vi "TestiLabviewLIVELowLevelv3 - Copy.vi"() -> ()   [LabVIEW 2018]
uses:
  <vilib>/myRIO/Instrument Drivers/Onboard IO/PWM/typedefs/PWM Reference.ctl
  <vilib>/myRIO/Common/Instrument Driver Framework/Utilities/typedefs/myRIO Generic Hardware Reference.ctl
  <vilib>/myRIO/Common/Instrument Driver Framework/Utilities/typedefs/Hardware Version Enum.ctl
  <vilib>/myRIO/Common/Instrument Driver Framework/Utilities/typedefs/myRIO v1.0 Reference.ctl
  <vilib>/myRIO/Common/Instrument Driver Framework/Utilities/typedefs/Generic FPGA Reference.ctl
  <vilib>/myRIO/Common/Instrument Driver Framework/myRIO v1.0/PWM/typedefs/PWM Channels Enum.ctl
  <vilib>/myRIO/Instrument Drivers/Onboard IO/PWM/typedefs/PWM Configuration.ctl
  <vilib>/userdefined/High Color/nirio_resource_hc.ctl
  <vilib>/vision/Image Controls.llb/IMAQ Image.ctl
  <vilib>/myRIO/Common/Instrument Driver Framework/myRIO v1.0/PWM/vis/myRIO v1.1 Open PWM.vi
  <vilib>/myRIO/Common/Instrument Driver Framework/Utilities/vis/Validate Channels.vi
  <vilib>/myRIO/Common/Instrument Driver Framework/myRIO v1.0/PWM/vis/myRIO v1.0 Reserve PWM.vi
  <vilib>/myRIO/Common/Instrument Driver Framework/myRIO v1.0/UART/vis/myRIO v1.0 Close UART.vi
  <vilib>/myRIO/Common/Instrument Driver Framework/myRIO v1.0/PWM/vis/myRIO v1.0 Build MUX Configuration PWM.vi
  <vilib>/myRIO/Common/Instrument Driver Framework/myRIO v1.0/Resource Manager/vis/myRIO v1.0 Reserve Channel List.vi
  <vilib>/myRIO/Common/Instrument Driver Framework/myRIO v1.0/Resource Manager/vis/myRIO v1.0 Create Configuration List.vi
  <vilib>/myRIO/Common/Instrument Driver Framework/myRIO v1.0/Resource Manager/vis/myRIO v1.0 Reserve Channel.vi
  <vilib>/myRIO/Common/Instrument Driver Framework/myRIO v1.0/Resource Manager/vis/myRIO v1.0 Unreserve Channel.vi
  <vilib>/myRIO/Common/Instrument Driver Framework/myRIO v1.0/Resource Manager/vis/myRIO v1.0 Build Mutex Name.vi
  <vilib>/Utility/VariantDataType/GetNumericInfo.vi
  <vilib>/Utility/error.llb/Error Cluster From Error Code.vi
  <vilib>/myRIO/Common/Instrument Driver Framework/myRIO v1.0/myRIO v1.1 Open.vi
  <vilib>/myRIO/Common/Instrument Driver Framework/Utilities/vis/IO Manager.vi
  <vilib>/myRIO/Common/Instrument Driver Framework/Utilities/vis/Configuration Manager.vi
  <vilib>/myRIO/Common/Instrument Driver Framework/myRIO v1.0/Resource Manager/vis/myRIO v1.0 Configure IO.vi
  <vilib>/myRIO/Common/Instrument Driver Framework/myRIO v1.0/myRIO v1.0 Close.vi
  <vilib>/myRIO/Common/Instrument Driver Framework/myRIO v1.0/PWM/vis/myRIO v1.0 Write PWM.vi
  <vilib>/myRIO/Common/Instrument Driver Framework/Utilities/vis/FPGA Ref Manager.vi
  <vilib>/myRIO/Common/Instrument Driver Framework/myRIO v1.0/myRIO v1.0 Reset FPGA.vi
  <vilib>/myRIO/Common/Instrument Driver Framework/myRIO v1.0/IRQ/vis/myRIO v1.0 IRQ Info FGV.vi
  <vilib>/myRIO/Common/Instrument Driver Framework/myRIO v1.0/IRQ/vis/myRIO v1.0 Timer IRQ Info FGV.vi
  <vilib>/myRIO/Common/Instrument Driver Framework/myRIO v1.0/IRQ/vis/myRIO v1.0 ISR Agent.vi
  <vilib>/myRIO/Instrument Drivers/Onboard IO/PWM/vis/myRIO PWM Open.xnode
  <vilib>/myRIO/Instrument Drivers/Onboard IO/PWM/PWM.lvlib
  <vilib>/myRIO/Instrument Drivers/Utilities/Utilities.lvlib
  <vilib>/vision/driver/NI_Vision_Acquisition_Software.lvlib
  <vilib>/vision/NI_Vision_Development_Module.lvlib
panel:
  in  "Number of Erosion (Advanced Morphology 1)":i32=12
  in  "Structuring Element (Basic Morphology 1) 2":i32[][](array[numeric])=[[0, 1, 0], [1, 1, 1], [0, 1, 0]]
  in  "Range (Threshold 1) 2":cluster{"Lower value":sgl, "Upper value":sgl}={"Lower value"=230.0, "Upper value"=255.0}
  in  "Color Plane (Color Plane Extraction 1) 2":i32(ring)=1 items=["Red", "Green", "Blue", "Hue", "Saturation", "Luminance", "Value", "Intensity"]
  in  "logfile base name":string="logfile"
  out "logfile name":path
  out "Image 5":T1(plugin-control)
  out "Antal isbjerg 4":i32
  out "X 4":dbl[](array[numeric])
  out "Y 4":dbl[](array[numeric])
  in  "Stop":bool
  # "Tager isbjerge i rækkefølgen: y: 0 -> max"
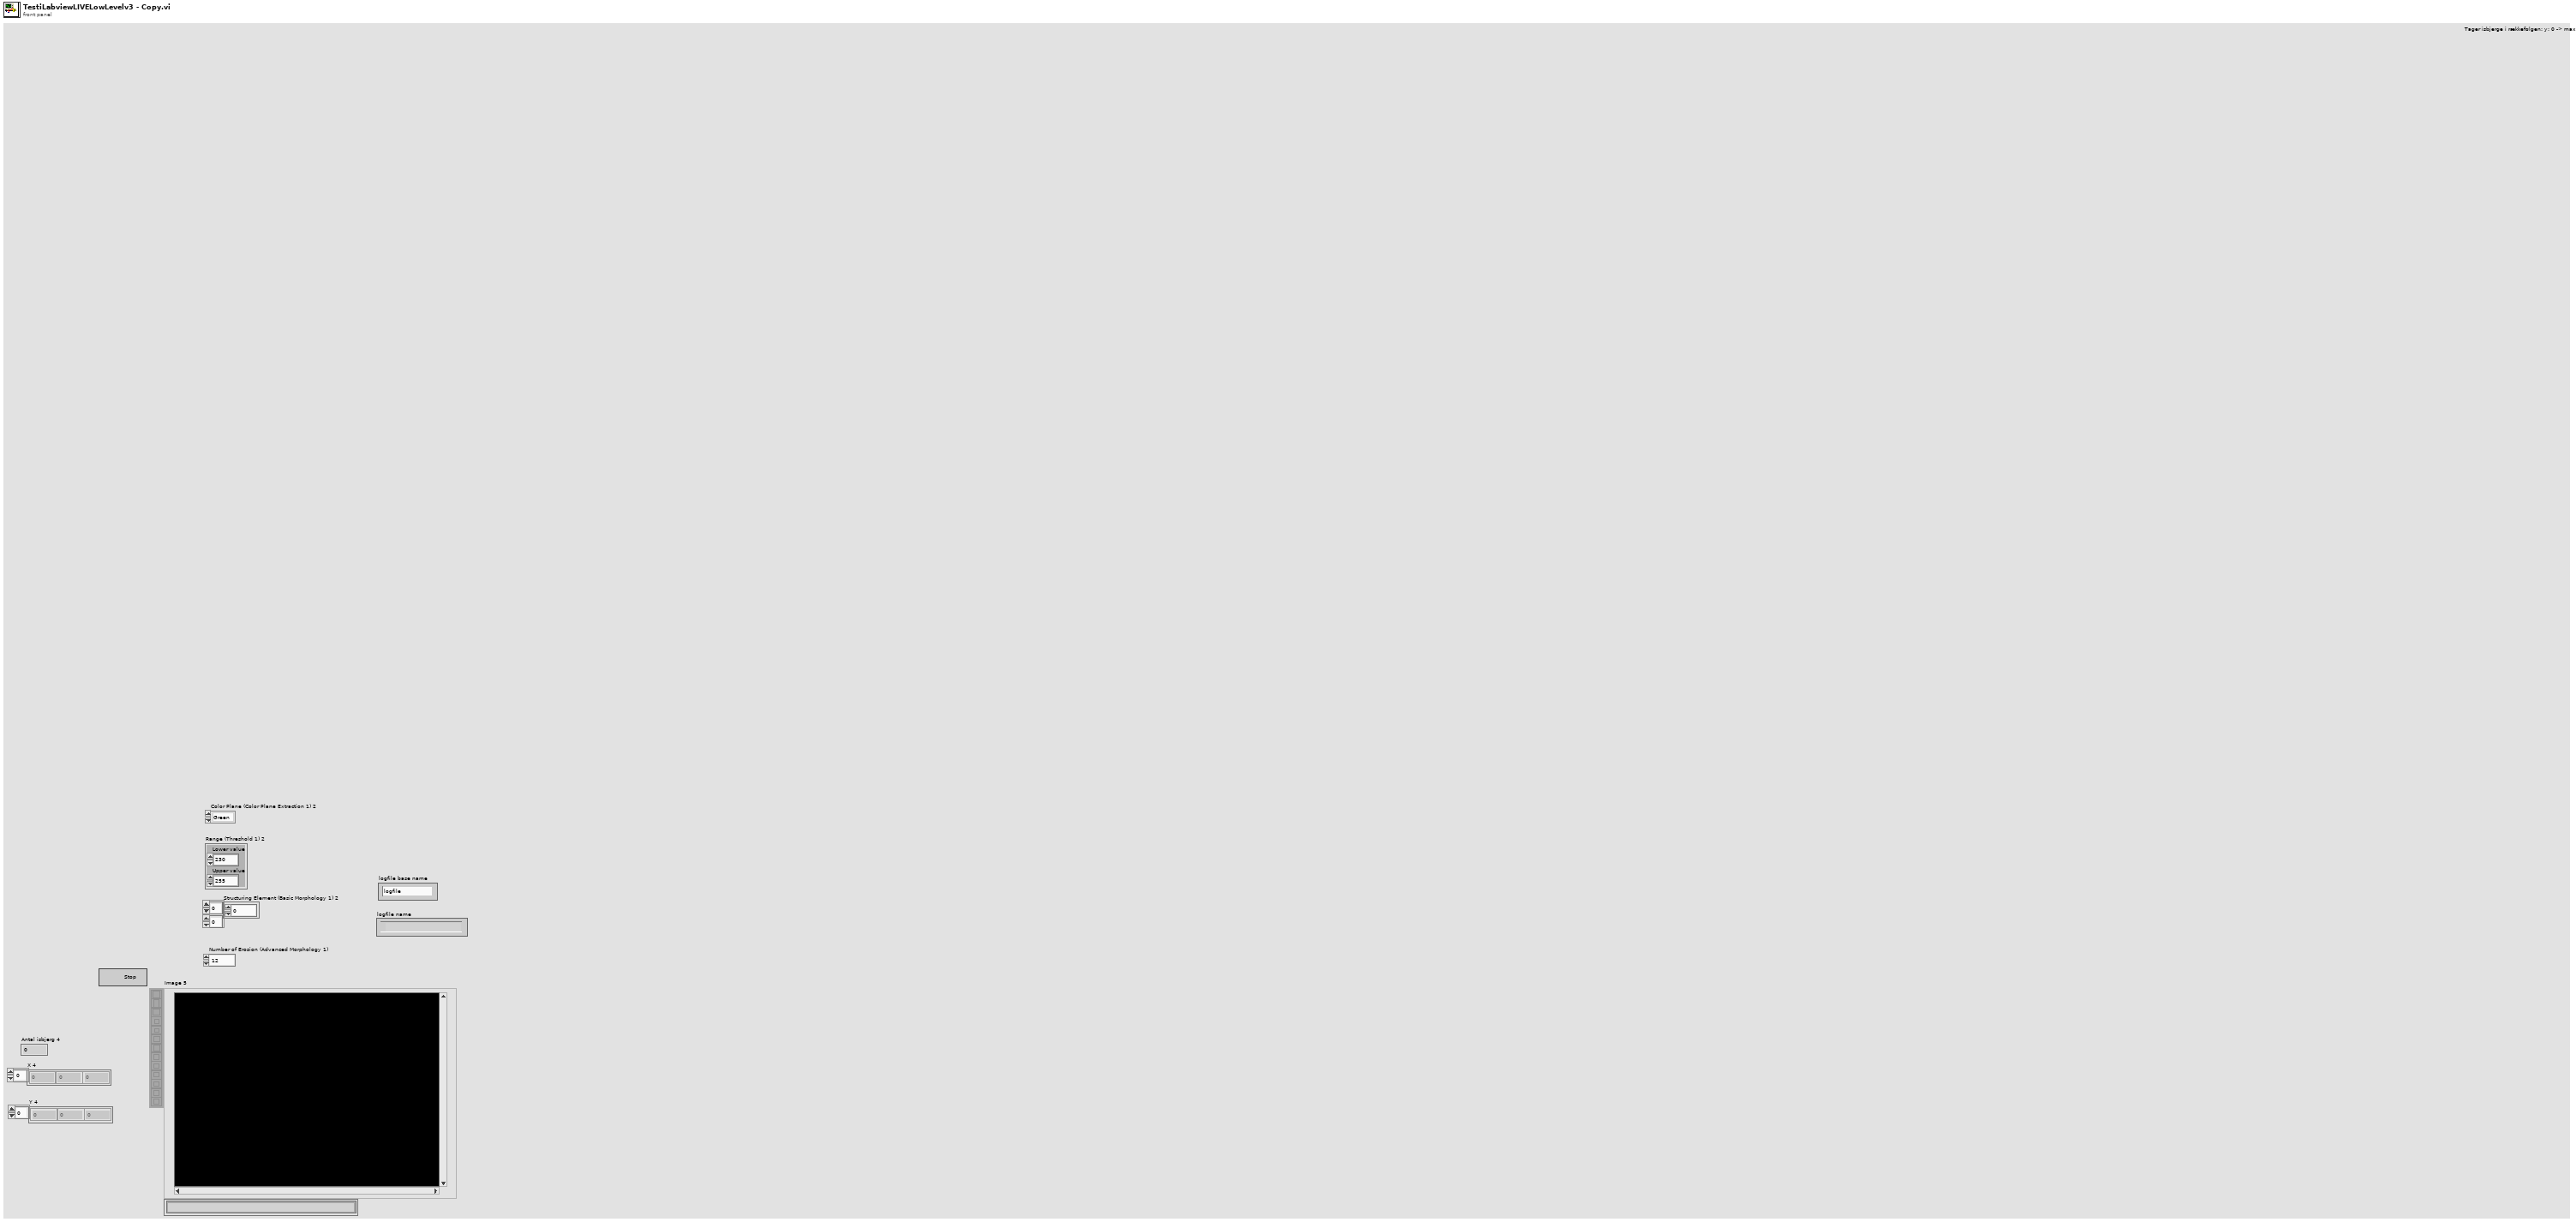
[diagram p1: front panel]
types:
  T1 = typedef "IMAQ Image.ctl" = refnum<image>
  T2 = typedef "nirio_resource_hc.ctl" = tag
  T3 = typedef "Hardware Version Enum.ctl" = enum16{"Unknown", "myRIO-1900", "myRIO-1950", "roboRIO", "NI ELVIS RIO CM", "ELVIS III"}
  T4 = enum32{"AutoM", "Close", "Dilate", "Erode", "Gradient", "Gradient out", "Gradient in", "Hit miss", "Open", "PClose", "POpen", "Thick", "Thin"}
  T5 = typedef "PWM.lvlib/PWM Reference.ctl" = cluster{"myRIO Reference":T6, "PWM Channels Enum":T9, "PWM Configuration":T10}
  T6 = typedef "myRIO Generic Hardware Reference.ctl" = cluster{"myRIO Model":T3, "myRIO Hardware Reference":T7}
  T7 = typedef "myRIO v1.0 Reference.ctl" = cluster{"Generic FPGA Reference":T8, "Allow multiple opens":bool}
  T8 = typedef "Generic FPGA Reference.ctl" = refnum<k20>
  T9 = typedef "PWM Channels Enum.ctl" = enum16{"Not Connected", "C/PWM0", "C/PWM1", "A/PWM0", "A/PWM1", "A/PWM2", "A/PWM3", "A/PWM4", "A/PWM5", "A/PWM6", "A/PWM7", "A/PWM8", "A/PWM9", "A/PWM10", "A/PWM11", "A/PWM12", "A/PWM13", "A/PWM14", "A/PWM15", "A/PWM16", "A/PWM17", "A/PWM18", "A/PWM19", "B/PWM0", "B/PWM1", "B/PWM2", "B/PWM3", "B/PWM4", "B/PWM5", "B/PWM6", "B/PWM7", "B/PWM8", "B/PWM9", "B/PWM10", "B/PWM11", "B/PWM12", "B/PWM13", "B/PWM14", "B/PWM15", "B/PWM16", "B/PWM17", "B/PWM18", "B/PWM19", "PWM/PWM0", "PWM/PWM1", "PWM/PWM2", "PWM/PWM3", "PWM/PWM4", "PWM/PWM5", "PWM/PWM6", "PWM/PWM7", "PWM/PWM8", "PWM/PWM9"}
  T10 = typedef "PWM.lvlib/PWM Configuration.ctl" = cluster{"Frequency":dbl, "Duty Cycle":dbl}
  T11 = typedef "Image Type" = u32
  T12 = typedef "IMAQdx.ctl" = refnum<k21>
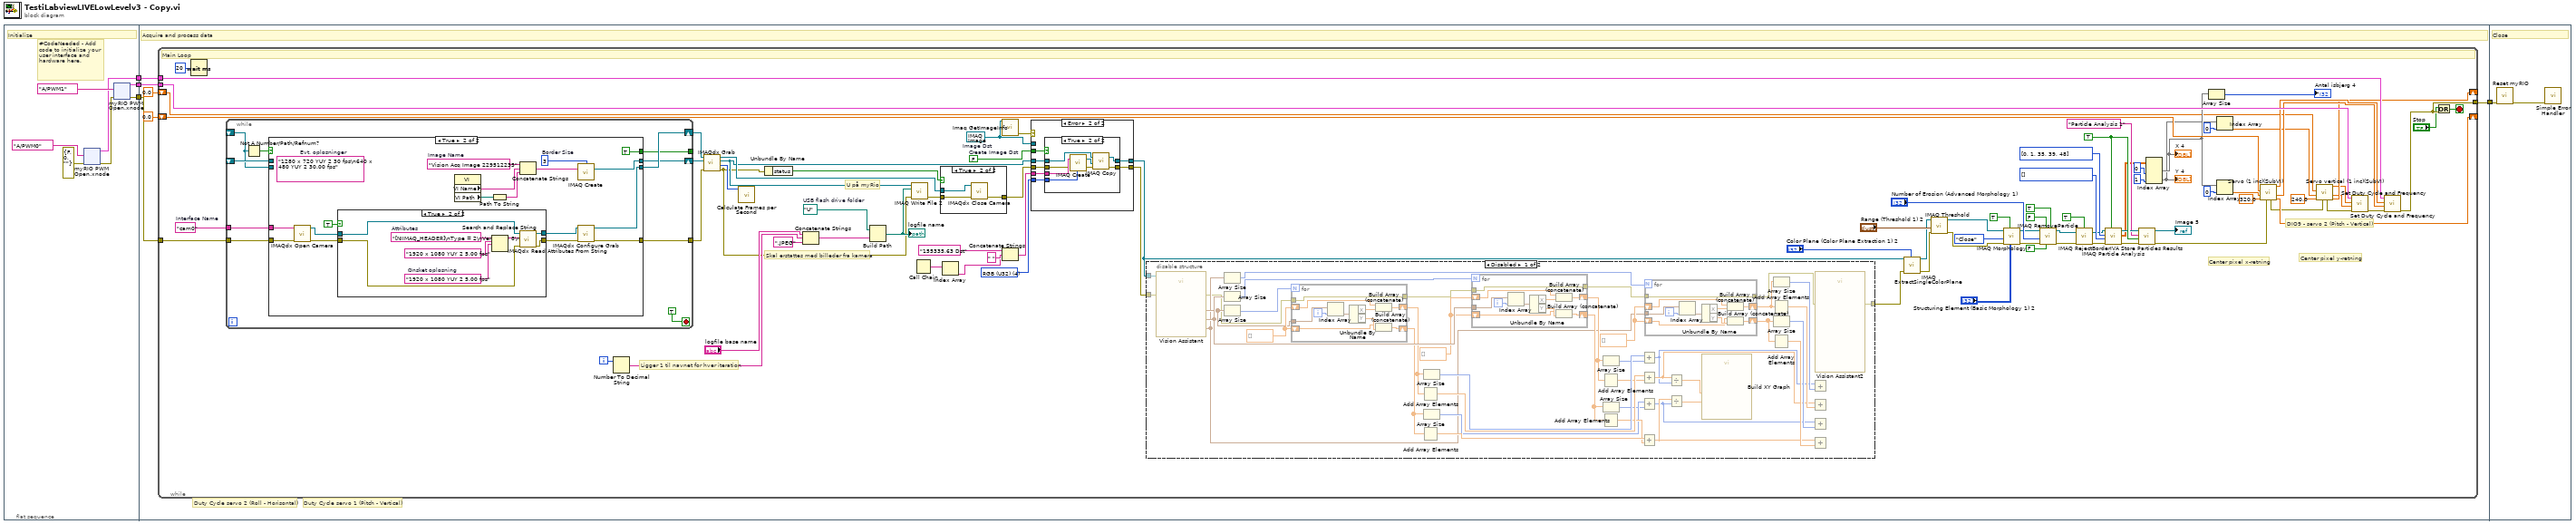
[diagram p0: block diagram]
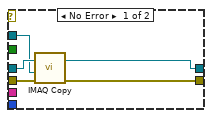
[diagram p6: hidden frame]
diagram:
  n1 = flat-sequence {
    tunnel: [w11] -> w4
    tunnel: [w10] -> w3
    tunnel: [w7] -> w2
    tunnel: w4 -> [w49]
    tunnel: w3 -> [w44]
    tunnel: w2 -> [w48]
    tunnel: [w47] -> w1
    tunnel: w1 -> [w278]
    frame #0 {
      # "#CodeNeeded - Add code to initialize your user interface and hardware here."
      # "Initialize"
      n2 = xnode "myRIO PWM Open.xnode"("error in (no error)"=errorcluster {"status"=FALSE, "code"=0, "source"=""} ("error in"), "Channel Name"=tag "A/PWM0") -> ("error out"=w5:errorcluster, "PWM Ref Out"=w7:T5)  [unwired: 1 in]
      n3 = xnode "myRIO PWM Open.xnode"("error in (no error)"=w5, "Channel Name"=tag "A/PWM1") -> ("error out"=w10:errorcluster, "PWM Ref Out"=w11:T5)  [unwired: 1 in]
    }
    frame #1 {
      # "Duty Cycle servo 2 (Roll - Horisontal)"
      # "Duty Cycle servo 1 (Pitch - Vertical)"
      # "Acquire and process data"
      n4 = while {
        tunnel: w49 -> [w137]
        tunnel: w48 -> [w136]
        tunnel: [w135] -> w47
        shift-right: [w94] -> _
        shift-left: 0.0 ("Duty Cycle servo 1 (Yaw - Horisontal)") -> [w98]
        shift-right: [w113] -> _
        shift-left: 0.0 ("Duty Cycle servo 1 (Yaw - Horisontal)") -> [w115]
        tunnel: w44 -> [w116]
        i -> [w82]
        stop <- w134 stop-if-true
        w60 = i32[] [] items=["Center of Mass X", "Center of Mass Y", "First Pixel X", "First Pixel Y", "Bounding Rect Left", "Bounding Rect Top", "Bounding Rect Right", "Bounding Rect Bottom", "Max Feret Diameter Start X", "Max Feret Diameter Start Y", "Max Feret Diameter End X", "Max Feret Diameter End Y", "Max Horiz. Segment Length Left", "Max Horiz. Segment Length Right", "Max Horiz. Segment Length Row", "-", "Bounding Rect Width", "Bounding Rect Height", "Bounding Rect Diagonal", "Perimeter", "Convex Hull Perimeter", "Holes' Perimeter", "Max Feret Diameter", "Equivalent Ellipse Major Axis", "Equivalent Ellipse Minor Axis", "Equivalent Ellipse Minor Axis (Feret)", "Equivalent Rect Long Side", "Equivalent Rect Short Side", "Equivalent Rect Diagonal", "Equivalent Rect Short Side (Feret)", "Average Horiz. Segment Length", "Average Vert. Segment Length", "Hydraulic Radius", "Waddel Disk Diameter", "-", "Area", "Holes' Area", "Particle & Holes' Area", "Convex Hull Area", "Image Area", "-", "Number of Holes", "Number of Horiz. Segments", "Number of Vert. Segments", "-", "Orientation", "Max Feret Diameter Orientation", "-", "% Area/Image Area", "% Area/(Particle & Holes' Area)", "Ratio of Equivalent Ellipse Axes", "Ratio of Equivalent Rect Sides", "-", "Elongation Factor", "Compactness Factor", "Heywood Circularity Factor", "Type Factor", "-", "Sum X", "Sum Y", "Sum XX", "Sum XY", "Sum YY", "Sum XXX", "Sum XXY", "Sum XYY", "Sum YYY", "-", "Moment of Inertia XX", "Moment of Inertia XY", "Moment of Inertia YY", "Moment of Inertia XXX", "Moment of Inertia XXY", "Moment of Inertia XYY", "Moment of Inertia YYY", "Norm. Moment of Inertia XX", "Norm. Moment of Inertia XY", "Norm. Moment of Inertia YY", "Norm. Moment of Inertia XXX", "Norm. Moment of Inertia XXY", "Norm. Moment of Inertia XYY", "Norm. Moment of Inertia YYY", "Hu Moment 1", "Hu Moment 2", "Hu Moment 3", "Hu Moment 4", "Hu Moment 5", "Hu Moment 6", "Hu Moment 7"] ("Real-World Measurements")
        w61 = i32[] [0, 1, 35, 39, 48] items=["Center of Mass X", "Center of Mass Y", "First Pixel X", "First Pixel Y", "Bounding Rect Left", "Bounding Rect Top", "Bounding Rect Right", "Bounding Rect Bottom", "Max Feret Diameter Start X", "Max Feret Diameter Start Y", "Max Feret Diameter End X", "Max Feret Diameter End Y", "Max Horiz. Segment Length Left", "Max Horiz. Segment Length Right", "Max Horiz. Segment Length Row", "-", "Bounding Rect Width", "Bounding Rect Height", "Bounding Rect Diagonal", "Perimeter", "Convex Hull Perimeter", "Holes' Perimeter", "Max Feret Diameter", "Equivalent Ellipse Major Axis", "Equivalent Ellipse Minor Axis", "Equivalent Ellipse Minor Axis (Feret)", "Equivalent Rect Long Side", "Equivalent Rect Short Side", "Equivalent Rect Diagonal", "Equivalent Rect Short Side (Feret)", "Average Horiz. Segment Length", "Average Vert. Segment Length", "Hydraulic Radius", "Waddel Disk Diameter", "-", "Area", "Holes' Area", "Particle & Holes' Area", "Convex Hull Area", "Image Area", "-", "Number of Holes", "Number of Horiz. Segments", "Number of Vert. Segments", "-", "Orientation", "Max Feret Diameter Orientation", "-", "% Area/Image Area", "% Area/(Particle & Holes' Area)", "Ratio of Equivalent Ellipse Axes", "Ratio of Equivalent Rect Sides", "-", "Elongation Factor", "Compactness Factor", "Heywood Circularity Factor", "Type Factor", "-", "Sum X", "Sum Y", "Sum XX", "Sum XY", "Sum YY", "Sum XXX", "Sum XXY", "Sum XYY", "Sum YYY", "-", "Moment of Inertia XX", "Moment of Inertia XY", "Moment of Inertia YY", "Moment of Inertia XXX", "Moment of Inertia XXY", "Moment of Inertia XYY", "Moment of Inertia YYY", "Norm. Moment of Inertia XX", "Norm. Moment of Inertia XY", "Norm. Moment of Inertia YY", "Norm. Moment of Inertia XXX", "Norm. Moment of Inertia XXY", "Norm. Moment of Inertia XYY", "Norm. Moment of Inertia YYY", "Hu Moment 1", "Hu Moment 2", "Hu Moment 3", "Hu Moment 4", "Hu Moment 5", "Hu Moment 6", "Hu Moment 7"] ("Pixel Measurements")
        w58 = TRUE ("Connectivity 4/8 (8)")
        w81 = path "U:/"  # USB flash drive folder
        w123 = "cam0"  # Interface Name
        w133 = T1 refnum  # Image Dst
        w125 = T11 4 items=["Grayscale (U8)", "Grayscale (I16)", "Grayscale (SGL)", "Complex (CSG)", "RGB (U32)", "HSL (U32)", "RGB (U64)", "Grayscale (U16)"] ("Image Dst Type")
        w131 = FALSE  # Create Image Dst
        # "U på myRio"
        # "Ligger 1 til navnet for hver iteration"
        # "Skal erstattes med billeder fra kamera"
        # "Center pixel y-retning"
        # "Center pixel x-retning"
        # "DIO9 - servo 2 (Pitch - Vertical)"
        # "Main Loop"
        n5 = Wait (ms)(milliseconds to wait=u32 20) -> ()  [unwired: 1 out]
        n6 = while "While Loop_template0" {
          shift-right: [w225] -> w118
          shift-left: _ -> [w218]
          tunnel: [w224] -> w124
          tunnel: w116 -> [w223]
          shift-right: [w221] -> w119
          shift-left: _ -> [w220]
          tunnel: w123 -> [w219]
          tunnel: [w216] -> _
          stop <- TRUE ("_template0") stop-if-true
          n7 = Not A Number/Path/Refnum?(number/path/refnum=w218) -> (NaN/Path/Refnum?=w217:bool)
          n8 = case "Case Structure_template0" shown="True" w217 {
            tunnel: [w228 w244] -> w225
            tunnel: w218 -> [w228 _]
            tunnel: [w227 w243] -> w224
            tunnel: w223 -> [w227 w245]
            tunnel: [w226 w242] -> w221
            tunnel: w220 -> [w226 _]
            tunnel: w219 -> [_ w232]
            tunnel: [_ TRUE] -> w216
            frame False {
            }
            frame True {
              (unwired) "1280 x 720 YUY 2 30 fps\n640 x 480 YUY 2 30.00 fps"  # Evt. opløsninger
              w229 = 3  # Border Size
              w237 = "Vision Acq Image 229512235"  # Image Name
              n9 = call <vilib>:"IMAQdx Open Camera.vi"("error in"=w245, "Session In"=w232) -> ("error out"=w235:errorcluster, "Session Out"=w236:T12)  [unwired: 1 in, 7 out]
              n10 = case shown="True" TRUE ("Init Attributes") {
                tunnel: w236 -> [w247 w255]
                tunnel: w235 -> [w246 w254]
                tunnel: [w247 w253] -> w234
                tunnel: [w246 w252] -> w233
                frame False {
                }
                frame True {
                  w248 = "1920 x 1080 YUY 2 5.00 fps"  # Ønsket opløsning
                  w251 = "[NIIMAQ_HEADER]\nType = 2\nVersion = 8\n\n[CAMERA_DATA]\nAcquisitionAttributes::Bayer::Algorithm = \"Bilinear\"\nAcquisitionAttributes::Bayer::GainB = \"1\"\nAcquisitionAttributes::Bayer::GainG = \"1\"\nAcquisitionAttributes::Bayer::GainR = \"1\"\nAcquisitionAttributes::Bayer::Pattern = \"Use hardware value\"\nAcquisitionAttributes::BitsPerPixel = \"Use hardware value\"\nAcquisitionAttributes::HardwareMaximumQueuedBufferCount = \"1000\"\nAcquisitionAttributes::HardwareRequeueBufferListThreshold = \"50\"\nAcquisitionAttributes::IgnoreFirstFrame = \"false\"\nAcquisitionAttributes::ImageDecoderCopyMode = \"Auto\"\nAcquisitionAttributes::OutputImageType = \"Auto\"\nAcquisitionAttributes::OverwriteMode = \"Get Newest\"\nAcquisitionAttributes::PixelSignedness = \"Use hardware value\"\nAcquisitionAttributes::ReceiveTimestampMode = \"None\"\nAcquisitionAttributes::ShiftPixelBits = \"false\"\nAcquisitionAttributes::SwapPixelBytes = \"false\"\nAcquisitionAttributes::Timeout = \"5000\"\nAcquisitionAttributes::VideoMode = \"1920 x 1080 YUY 2 5.00 fps\"\nCameraAttributes::BacklightCompensation::Mode = \"Manual\"\nCameraAttributes::BacklightCompensation::Value = \"0\"\nCameraAttributes::Brightness::Mode = \"Manual\"\nCameraAttributes::Brightness::Value = \"168\"\nCameraAttributes::Contrast::Mode = \"Manual\"\nCameraAttributes::Contrast::Value = \"5\"\nCameraAttributes::Exposure::Mode = \"AutoAperaturePriority\"\nCameraAttributes::Focus::Mode = \"Auto\"\nCameraAttributes::Pan::Mode = \"Manual\"\nCameraAttributes::Pan::Value = \"0\"\nCameraAttributes::PowerLineFrequency::Mode = \"60Hz\"\nCameraAttributes::Saturation::Mode = \"Manual\"\nCameraAttributes::Saturation::Value = \"103\"\nCameraAttributes::Sharpness::Mode = \"Manual\"\nCameraAttributes::Sharpness::Value = \"25\"\nCameraAttributes::Tilt::Mode = \"Manual\"\nCameraAttributes::Tilt::Value = \"0\"\nCameraAttributes::WhiteBalance::Mode = \"Auto\"\nCameraAttributes::Zoom::Mode = \"Manual\"\nCameraAttributes::Zoom::Value = \"0\"\n"  # Attributes
                  n11 = Search and Replace String(input string=w251, search string="1920 x 1080 YUY 2 5.00 fps", replace string=w248) -> (result string=w249:string)  [unwired: 5 in, 3 out]
                  n12 = call <vilib>:"IMAQdx Read Attributes From String.vi"("error in"=w254, "Attributes String In"=w249, "Session In"=w255) -> ("error out"=w252:errorcluster, "Session Out"=w253:T12)  [unwired: 7 out]
                }
              }
              n13 = property class="VI"() -> ("VI Name"=w240:string, "VI Path"=w241:path)  [unwired: 2 in, 2 out]
              n14 = Path To String(path=w241) -> (string=w239:string)
              n15 = Concatenate Strings(w237, w240, w239) -> (w238:string)
              n16 = call "IMAQ Create"("Border Size"=w229, "Image Name"=w238) -> ("New Image"=w242:T1)  [unwired: 2 in, 2 out]
              n17 = call <vilib>:"IMAQdx Configure Grab.vi"("error in"=w233, "Session In"=w234) -> ("error out"=w243:errorcluster, "Session Out"=w244:T12)  [unwired: 8 out]
            }
          }
        }
        n18 = Number To Decimal String(number=w82) -> (decimal integer string=w87:string)  [unwired: 1 in]
        n19 = call <vilib>:"IMAQdx Grab.vi"("error in"=w124, "Image In"=w119, "Session In"=w118) -> ("error out"=w84:errorcluster, "Buffer Number Out"=w122:u32, "Image Out"=w85:T1, "Session Out"=w121:T12)  [unwired: 1 in, 4 out]
        n20 = call <vilib>:"Calculate Frames per Second.vi"("Buffer Number"=w122) -> ()  [unwired: 2 in, 9 out]
        n21 = Unbundle By Name(w84) -> ("status"=w107:bool)
        n22 = Concatenate Strings "Concatenate Strings"("logfile base name", w87, ".JPEG" ("string")) -> (w89:string)
        n23 = Build Path(base path=w81, name or relative path=w89) -> (appended path=w90:path)
        "logfile name" <- w90
        n24 = call-poly "IMAQ Write File 2"("error in (no error)"=w84, "File Path"=w90, "Image"=w85) -> ("error out"=w83:errorcluster)  [unwired: 7 in, 1 out]
        n25 = Call Chain() -> (call chain=w130:string[])
        n26 = case "Case Structure_template1" shown="True" w107 {
          tunnel: [w212 w214] -> w120
          tunnel: w83 -> [w212 w215]
          tunnel: w121 -> [_ w213]
          frame False {
          }
          frame True {
            n27 = call <vilib>:"IMAQdx Close Camera.vi"("error in"=w215, "Session In"=w213) -> ("error out"=w214:errorcluster)  [unwired: 9 out]
          }
        }
        n28 = Index Array(array=w130) -> (element=w128:string)  [unwired: 1 in]
        n29 = call "Imaq GetImageInfo"("Image"=w133) -> ("error out"=w132:errorcluster)  [unwired: 1 in, 9 out]
        n30 = Concatenate Strings("155335,63 Dst" ("Image Dst Name"), " ", w128) -> (w126:string)
        n31 = case shown="Error" w132 {
          tunnel: [w260 w264] -> w52
          tunnel: [w259 w263] -> w117
          tunnel: w85 -> [w258 w265]
          tunnel: w120 -> [w257 w261]
          tunnel: w133 -> [w256 _]
          tunnel: w126 -> [_ w267]
          tunnel: w125 -> [_ w266]
          tunnel: w131 -> [_ w262]
          frame No Error {
            n32 = call "IMAQ Copy"("error in (no error)"=w257, "Image Dst"=w256, "Image Src"=w258) -> ("error out"=w259:errorcluster, "Image Dst Out"=w260:T1)  [unwired: 3 out]
          }
          frame Error {
            n33 = case shown="True" w262 {
              tunnel: w267 -> [_ w277]
              tunnel: w266 -> [_ w276]
              tunnel: w265 -> [w269 w274]
              tunnel: [w269 w273] -> w264
              tunnel: [w268 w272] -> w263
              tunnel: w261 -> [w268 w270]
              frame False {
              }
              frame True {
                n34 = call "IMAQ Create"("Image Name"=w277, "Image Type"=w276, "error in (no error)"=w270) -> ("New Image"=w275:T1, "error out"=w271:errorcluster)  [unwired: 1 in, 1 out]
                n35 = call "IMAQ Copy"("error in (no error)"=w271, "Image Dst"=w275, "Image Src"=w274) -> ("error out"=w272:errorcluster, "Image Dst Out"=w273:T1)  [unwired: 3 out]
              }
            }
          }
        }
        n36 = disable-structure shown="Disabled" {
          disable-tunnel: w117 -> [w181 _]
          disable-tunnel: w52 -> [w142 _]
          disable-tunnel: [w138 _] -> w50
          frame Disabled {
            w161 = dbl[] []
            w174 = dbl[] []
            w178 = dbl[] []
            n37 = call "Vision Assistant"("Image In"=w142, "error in"=w181) -> ("Feature Points Coordinates (Feature Detection 3)"=w159:cluster{"X":dbl, "Y":dbl}[], "Feature Points Coordinates (Feature Detection 1)"=w163:cluster{"X":dbl, "Y":dbl}[], "Feature Points Coordinates (Feature Detection 2)"=w179:cluster{"X":dbl, "Y":dbl}[], "error out"=w153:errorcluster)  [unwired: 21 in, 1 out]
            n38 = Array Size(array=w159) -> (size(s)=w160:i32)
            n39 = Array Size(array=w179) -> (size(s)=w180:i32)
            n40 = Array Size(array=w163) -> (size(s)=w175:i32)
            n41 = for {
              N: w175 -> [_]
              shift-right: [w199] -> w173
              shift-left: w174 -> [w194]
              shift-right: [w198] -> w172
              shift-left: w174 -> [w195]
              tunnel: w163 -> [w193]
              tunnel: w153 -> [w192]
              tunnel: [w192] -> w152
              i -> [w201]
              n42 = Index Array(array=w193, index=w201) -> (element=w200:cluster{"X":dbl, "Y":dbl})
              n43 = Unbundle By Name(w200) -> ("X"=w197:dbl, "Y"=w196:dbl)
              n44 = Build Array (concatenate)(w194, w197) -> (w199:dbl[])
              n45 = Build Array (concatenate)(w195, w196) -> (w198:dbl[])
            }
            n46 = Add Array Elements(numeric array=w173) -> (sum=w169:dbl)
            n47 = Add Array Elements(numeric array=w172) -> (sum=w167:dbl)
            n48 = Array Size(array=w173) -> (size(s)=w171:i32)
            n49 = Array Size(array=w172) -> (size(s)=w165:i32)
            n50 = for {
              N: w180 -> [_]
              shift-right: [w209] -> w177
              shift-left: w178 -> [w204]
              shift-right: [w208] -> w176
              shift-left: w178 -> [w205]
              tunnel: w179 -> [w203]
              tunnel: w152 -> [w202]
              tunnel: [w202] -> w151
              i -> [w211]
              n51 = Index Array(array=w203, index=w211) -> (element=w210:cluster{"X":dbl, "Y":dbl})
              n52 = Unbundle By Name(w210) -> ("X"=w207:dbl, "Y"=w206:dbl)
              n53 = Build Array (concatenate)(w204, w207) -> (w209:dbl[])
              n54 = Build Array (concatenate)(w205, w206) -> (w208:dbl[])
            }
            n55 = Add Array Elements(numeric array=w177) -> (sum=w168:dbl)
            n56 = Add Array Elements(numeric array=w176) -> (sum=w166:dbl)
            n57 = Array Size(array=w177) -> (size(s)=w170:i32)
            n58 = Array Size(array=w176) -> (size(s)=w164:i32)
            n59 = Add(x=w171, y=w170) -> (x+y=w145:i32)
            n60 = Add(x=w169, y=w168) -> (x+y=w146:dbl)
            n61 = Add(x=w165, y=w164) -> (x+y=w143:i32)
            n62 = Add(x=w167, y=w166) -> (x+y=w144:dbl)
            n63 = for {
              N: w160 -> [_]
              shift-right: [w189] -> w162
              shift-left: w161 -> [w184]
              shift-right: [w188] -> w155
              shift-left: w161 -> [w185]
              tunnel: w159 -> [w183]
              tunnel: w151 -> [w182]
              tunnel: [w182] -> w150
              i -> [w191]
              n64 = Index Array(array=w183, index=w191) -> (element=w190:cluster{"X":dbl, "Y":dbl})
              n65 = Unbundle By Name(w190) -> ("X"=w187:dbl, "Y"=w186:dbl)
              n66 = Build Array (concatenate)(w184, w187) -> (w189:dbl[])
              n67 = Build Array (concatenate)(w185, w186) -> (w188:dbl[])
            }
            n68 = Divide(x=w146, y=w145) -> (x/y=w148:dbl)
            n69 = Divide(x=w144, y=w143) -> (x/y=w147:dbl)
            n70 = call "Build XY Graph"("Y Input"=w147, "X Input"=w148) -> ("XY Graph"=w149:cluster{"X":dbl[], "Y":dbl[]}[])  [unwired: 8 in, 1 out]
            n71 = Add Array Elements(numeric array=w162) -> (sum=w157:dbl)
            n72 = Add Array Elements(numeric array=w155) -> (sum=w156:dbl)
            n73 = Array Size(array=w162) -> (size(s)=w158:i32)
            n74 = Array Size(array=w155) -> (size(s)=w154:i32)
            n75 = Add(x=w145, y=w158) -> ()  [unwired: 1 out]
            n76 = Add(x=w146, y=w157) -> ()  [unwired: 1 out]
            n77 = Add(x=w143, y=w154) -> ()  [unwired: 1 out]
            n78 = Add(x=w144, y=w156) -> ()  [unwired: 1 out]
            n79 = call "Vision Assistant2"("error in"=w150) -> ("Color Plane (Color Plane Extraction 1)"=w139:i32, "Range (Threshold 1)"=w140:cluster{"Lower value":sgl, "Upper value":sgl}, "Structuring Element (Basic Morphology 1)"=w141:i32[][], "error out"=w138:errorcluster)  [unwired: 21 in, 2 out]
          }
          frame Enabled {
          }
        }
        n80 = call "IMAQ ExtractSingleColorPlane"("Color Plane"="Color Plane (Color Plane Extraction 1) 2", "error in (no error)"=w50, "Image Src"=w52) -> ("error out"=w79:errorcluster, "Image Dst Out"=w77:T1)  [unwired: 1 in, 6 out]
        n81 = call "IMAQ Threshold"("error in (no error)"=w79, "Range"="Range (Threshold 1) 2", "Image Src"=w77) -> ("error out"=w76:errorcluster, "Image Dst Out"=w72:T1)  [unwired: 3 in, 4 out]
        n82 = call "IMAQ Morphology"("Structuring Element"="Structuring Element (Basic Morphology 1) 2", "Square/Hexa (Square)"=TRUE, "error in (no error)"=w76, "Operation"=T4."Close", "Image Src"=w72) -> ("error out"=w71:errorcluster, "Image Dst Out"=w66:T1)  [unwired: 2 in, 3 out]
        n83 = call "IMAQ RemoveParticle"("Connectivity 4/8 (8)"=TRUE, "Low Pass/High Pass (Low)"=FALSE, "Square/Hexa (Square)"=FALSE, "error in (no error)"=w71, "Number of Erosion"="Number of Erosion (Advanced Morphology 1)", "Image Src"=w66) -> ("error out"=w65:errorcluster, "Image Dst Out"=w63:T1)  [unwired: 1 in, 3 out]
        n84 = call "IMAQ RejectBorder"("error in (no error)"=w65, "Image Src"=w63, "Connectivity 4/8 (8)"=TRUE) -> ("error out"=w62:errorcluster, "Image Dst Out"=w59:T1)  [unwired: 1 in, 2 out]
        n85 = call "IMAQ Particle Analysis"("Connectivity 4/8 (8)"=w58, "error in (no error)"=w62, "Real-World Measurements"=w60, "Pixel Measurements"=w61, "Image"=w59) -> ("error out"=w55:errorcluster, "Particle Measurements (Pixels)"=w51:dbl[][], "Image Out (duplicate)"=w57:T1)  [unwired: 4 out]
        n86 = call <vilib>:"IVA Store Particles Results.vi"("error in (no error)"=w55, "Connectivity 4/8 (8)"=w58, "Step Name"="Particle Analysis 1", "Image in"=w57) -> ("error out"=w53:errorcluster, "Image dup"=→"Image 5":T1)  [unwired: 6 out]
        n87 = Index Array(array=w51, index (col) #1=0 ("index (col)"), index (col) #2=1 ("index (col)")) -> (element #1=w102:dbl[], element #2=w99:dbl[])  [unwired: 2 in]
        "Y 4" <- w99
        "X 4" <- w102
        n88 = Array Size(array=w102) -> (size(s)=→"Antal isbjerg 4":i32)
        n89 = Index Array(array=w99, index=0) -> (element=w91:dbl)
        n90 = Index Array(array=w102, index=0) -> (element=w101:dbl)
        n91 = call "Servo (1 inc)(SubVI).vi"("error constant 2"=w53, "Center pixel"=320.0 ("Center pixel 2"), "Pixel value"=w101, "Position."=w115) -> ("Position 2"=w113:dbl, "freq [Hz]"=w114:dbl, "Duty"=w112:dbl, "error constant"=w96:errorcluster)  [unwired: 3 in, 1 out]
        n92 = call "Servo vertical (1 inc)(SubVI).vi"("error constant 2"=w96, "Center pixel"=240.0, "Pixel value"=w91, "Position."=w98) -> ("Position 2"=w94:dbl, "freq [Hz]"=w93:dbl, "Duty"=w92:dbl, "error constant"=w95:errorcluster)  [unwired: 3 in, 1 out]
        n93 = call <vilib>:"Set Duty Cycle and Frequency.vi"("error in (no error)"=w95, "Frequency [Hz]"=w93, "Duty Cycle"=w92, "PWM Ref In"=w137) -> ("error out"=w108:errorcluster)  [unwired: 5 in, 1 out]
        n94 = call <vilib>:"Set Duty Cycle and Frequency.vi"("error in (no error)"=w108, "Frequency [Hz]"=w114, "Duty Cycle"=w112, "PWM Ref In"=w136) -> ("error out"=w135:errorcluster)  [unwired: 5 in, 1 out]
        n95 = Or(x="Stop", y=w135) -> (x .or. y?=w134:bool)
      }
    }
    frame #2 {
      # "Close"
      n96 = call <vilib>:"Reset myRIO.vi"("error in (no error)"=w278) -> ("error out"=w279:errorcluster)  [unwired: 10 in]
      n97 = call <vilib>:"Simple Error Handler.vi"("error in (no error)"=w279) -> ()  [unwired: 4 in, 5 out]
    }
  }
